vi "Parse asset list.vi"(7 "Error in":errorcluster, 9 "Server URL":string, 10 "client handle":T1) -> (0 "error out":errorcluster, 2 "Array":string[][](array[string]), 3 "client handle out":T1)   [LabVIEW 2020]
uses:
  <vilib>/httpClient/ClientHandle.ctl
  <vilib>/httpClient/LabVIEWHTTPClient.lvlib
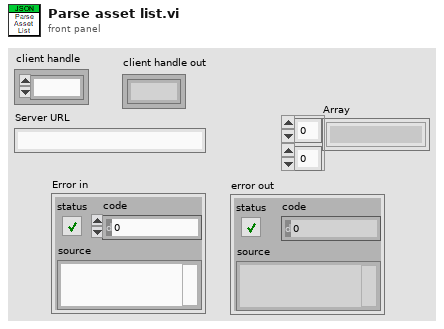
[diagram p1: front panel]
types:
  T1 = typedef "LabVIEWHTTPClient.lvlib/ClientHandle.ctl" = refnum<k1>
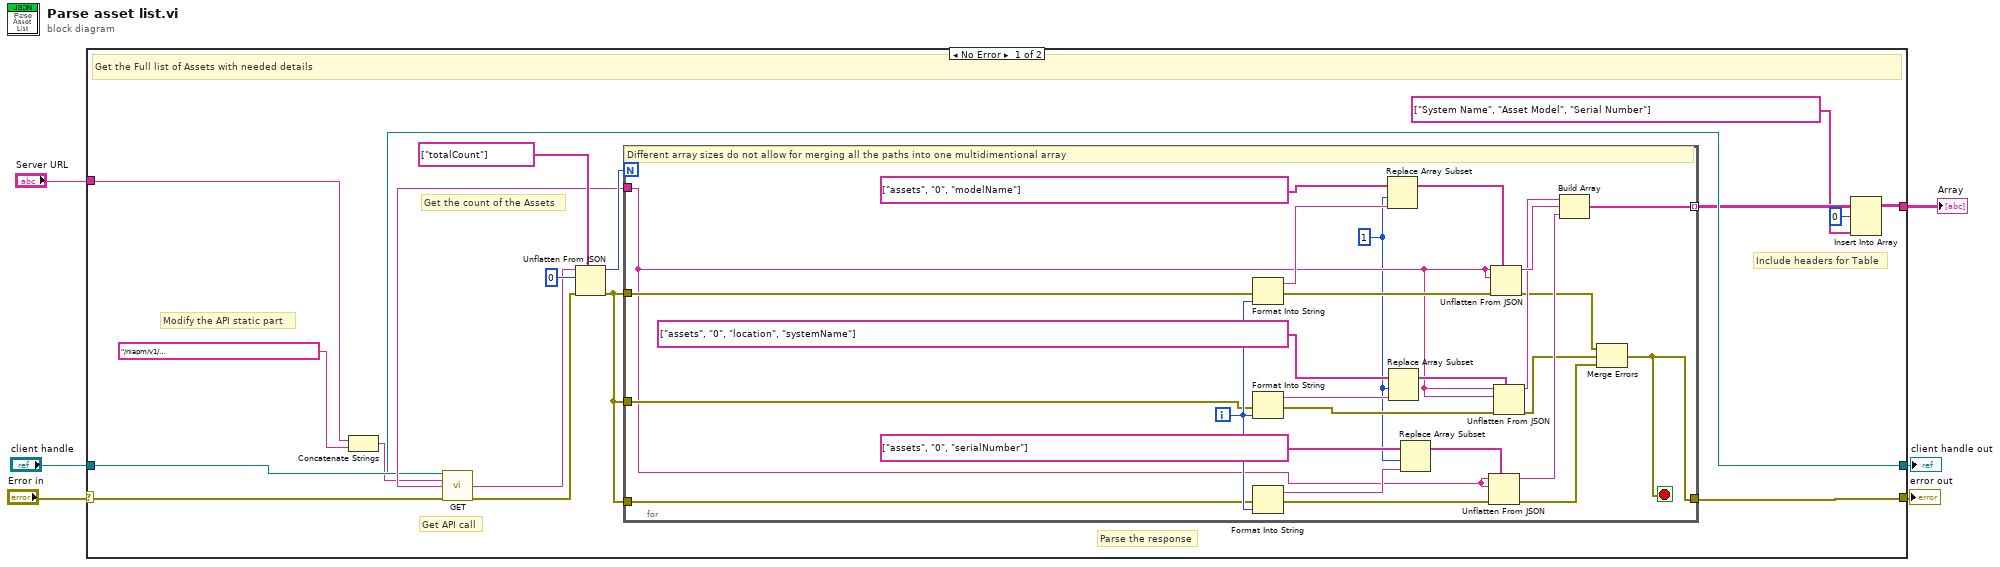
[diagram p0: block diagram]
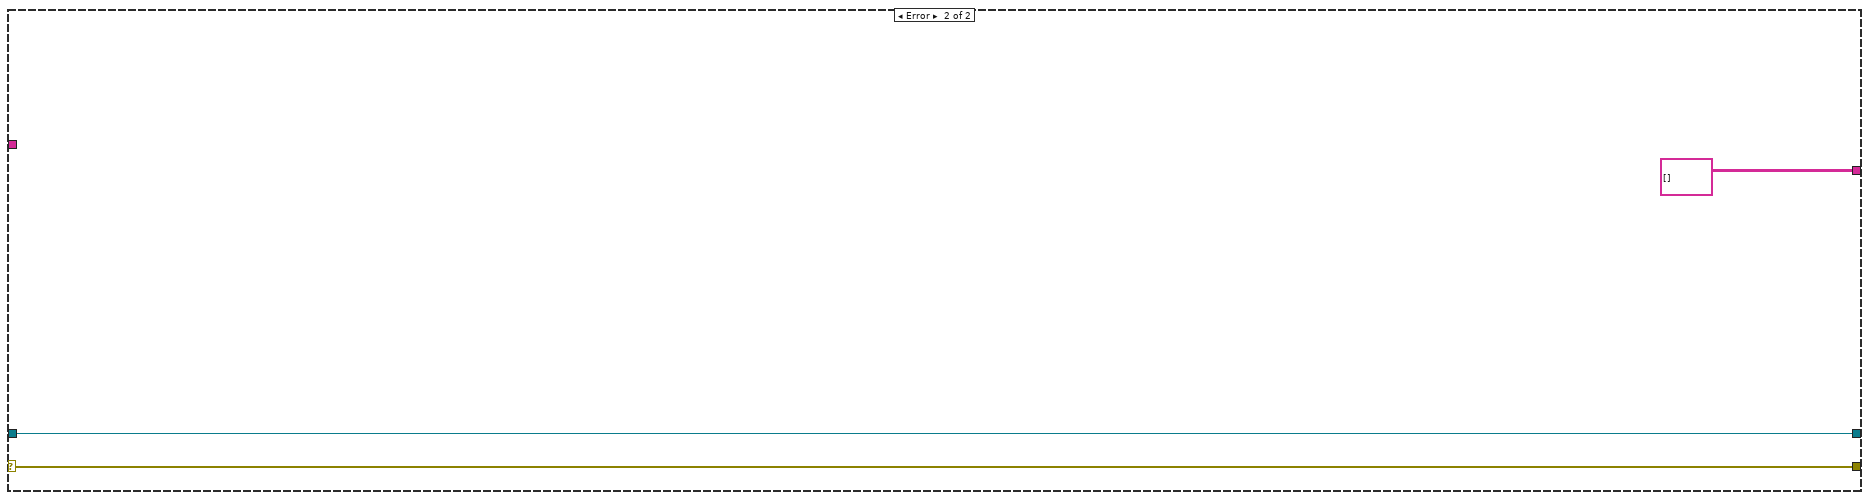
[diagram p2: hidden frame]
diagram:
  n1 = case shown="No Error" "Error in" {
    selector: "Error in" -> [w18 w52]
    tunnel: [w19 w52] -> w5
    tunnel: [w8 string[][] []] -> w4
    tunnel: "client handle" -> [w15 w50]
    tunnel: [w14 w50] -> w2
    tunnel: "Server URL" -> [w12 _]
    frame No Error {
      # "Include headers for Table"
      # "Parse the response"
      # "Get API call"
      # "Modify the API static part"
      # "Get the count of the Assets"
      # "Get the Full list of Assets with needed details"
      n2 = Concatenate Strings(w12, "/niapm/v1/assets?skip=0&take=-1&calibratableOnly=false&responseFormat=JSON&destination=INLINE&fileIngestionWorkspace=5bc5e9092a4fa4c71cfa7197" ("List of calibratable assets API")) -> (w11:string)
      n3 = call <vilib>:"GET.vi"("client handle"=w15, "url"=w11, "error in (no error)"=w18) -> ("client handle out"=w14:T1, "body"=w17:string, "error out"=w16:errorcluster)  [unwired: 9 in, 1 out]
      n4 = Unflatten From JSON(path=string[] ["totalCount"], JSON string=w17, type and defaults=0 ("index"), error in (no error)=w16) -> (value=w23:i32, error out=w20:errorcluster)  [unwired: 3 in]
      n5 = for {
        N: w23 -> [_]
        tunnel: w17 -> [w29]
        tunnel: [w41] -> w10 mode=indexing
        tunnel: w20 -> [w32]
        tunnel: w20 -> [w31]
        tunnel: w20 -> [w30]
        tunnel: [w24] -> w19
        i -> [w37]
        stop <- w24 stop-if-true
        w28 = 1 ("index")
        # "Different array sizes do not allow for merging all the paths into one multidimentional array"
        n6 = Format Into String(error in=w30, w37) -> (resulting string=w48:string, error out=w33:errorcluster)  [unwired: 2 in]
        n7 = Format Into String(error in=w31, w37) -> (resulting string=w45:string, error out=w34:errorcluster)  [unwired: 2 in]
        n8 = Format Into String(error in=w32, w37) -> (resulting string=w40:string, error out=w35:errorcluster)  [unwired: 2 in]
        n9 = Replace Array Subset(array=string[] ["assets", "0", "modelName"], new element=w48, index=w28) -> (w47:string[])
        n10 = Replace Array Subset(array=string[] ["assets", "0", "location", "systemName"], new element=w45, index=w28) -> (w46:string[])
        n11 = Replace Array Subset(array=string[] ["assets", "0", "serialNumber"], new element=w40, index=w28) -> (w39:string[])
        n12 = Unflatten From JSON(path=w39, JSON string=w29, type and defaults=w29, error in (no error)=w35) -> (value=w36:string, error out=w26:errorcluster)  [unwired: 3 in]
        n13 = Unflatten From JSON(path=w47, JSON string=w29, type and defaults=w29, error in (no error)=w33) -> (value=w43:string, error out=w25:errorcluster)  [unwired: 3 in]
        n14 = Unflatten From JSON(path=w46, JSON string=w29, type and defaults=w29, error in (no error)=w34) -> (value=w42:string, error out=w27:errorcluster)  [unwired: 3 in]
        n15 = Build Array(w42, w43, w36) -> (w41:string[])
        n16 = Merge Errors(w25, w27, w26) -> (w24:errorcluster)
      }
      n17 = Insert Into Array(array=w10, index (row)=0, new element=string[] ["System Name", "Asset Model", "Serial Number"]) -> (w8:string[][])  [unwired: 1 in]
    }
    frame Error {
    }
  }
  "error out" <- w5
  "Array" <- w4
  "client handle out" <- w2
